vi "Config_LoadCreate.vi"(7 "Config In":path, 8 "error In":errorcluster, 10 "Configuration Cluster":T1={"General"={"Config.ini"=path "", "Default Logging Path"=path ""}, "Hardware"={"Measure Rate (1/s)"=0, "HP DMM VISA"="", "LS 335 VISA"="", "HP DM"={"Range"=enum."Autorange", "Autozero"=FALSE, "Display"=enum."3 1/2 Digit", "Blank LCD"=FALSE}}, "Operation"={"Operation Mode"=enum."Idle-Off", "Status"="", "NewLog?"=FALSE, "OvenWarn"=FALSE}}) -> (0 "error out":errorcluster, 2 "Configuration Cluster Out":T1={"General"={"Config.ini"=path "", "Default Logging Path"=path ""}, "Hardware"={"Measure Rate (1/s)"=0, "HP DMM VISA"="", "LS 335 VISA"="", "HP DM"={"Range"=enum."Autorange", "Autozero"=FALSE, "Display"=enum."3 1/2 Digit", "Blank LCD"=FALSE}}, "Operation"={"Operation Mode"=enum."Idle-Off", "Status"="", "NewLog?"=FALSE, "OvenWarn"=FALSE}})   [LabVIEW 2021]
uses:
  Config_Cluster.ctl
  Mode_Enum.ctl
  <vilib>/Utility/config.llb/Read Key (Path).vi
  <vilib>/Utility/config.llb/NI_LVConfig.lvlib
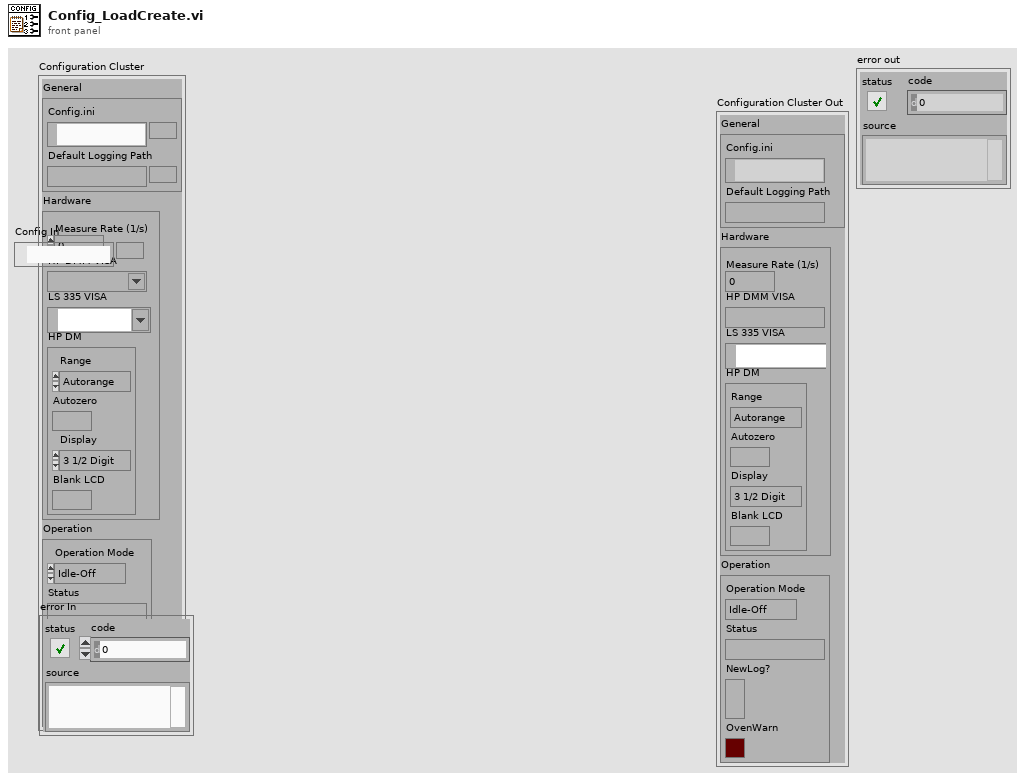
[diagram p1: front panel]
types:
  T1 = typedef "Config_Cluster.ctl" = cluster{"General":cluster{"Config.ini":path, "Default Logging Path":path}, "Hardware":cluster{"Measure Rate (1/s)":i32, "HP DMM VISA":refnum<visa-resource-name>, "LS 335 VISA":refnum<visa-resource-name>, "HP DM":cluster{"Range":enum16{"Autorange", "30mV", "300mV", "3V", "30V"}, "Autozero":bool, "Display":enum16{"3 1/2 Digit", "4 1/2 Digit", "5 1/2 Digit"}, "Blank LCD":bool}}, "Operation":cluster{"Operation Mode":T2, "Status":string, "NewLog?":bool, "OvenWarn":bool}}
  T2 = typedef "Mode_Enum.ctl" = enum16{"OvenNRDY", "Logging", "Idle-Off", "Idle"}
  T3 = typedef "NI_LVConfig.lvlib/Config Data RefNum.ctl" = refnum<k1>
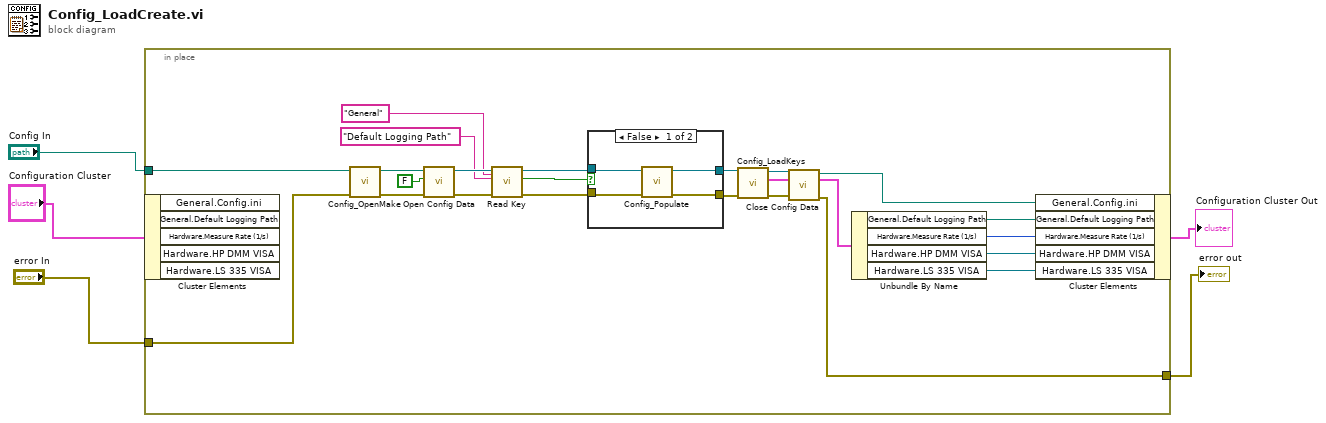
[diagram p0: block diagram]
diagram:
  n1 = in-place {
    in-place-border: "error In" -> [w27]
    in-place-border: "Config In" -> [w28]
    in-place-border: [w8] -> w1
    n2 = in-place-cluster #1("Configuration Cluster") -> ()  [unwired: 5 out]
    n3 = call "Config_OpenMake.vi"("error in (no error)"=w27, "Config Path"=w28) -> ("error out"=w24:errorcluster, "File Path"=w26:path)  [unwired: 8 in]
    n4 = call <vilib>:"Open Config Data.vi"("error in (no error)"=w24, "create file if necessary (T)"=FALSE, "configuration file path"=w26) -> ("error out"=w22:errorcluster, "refnum"=w23:T3)  [unwired: 6 in, 1 out]
    n5 = call-poly <vilib>:"Read Key.vi"("section"="General", "error in (no error)"=w22, "key"="Default Logging Path", "refnum"=w23) -> ("error out"=w18:errorcluster, "found?"=w17:bool, "refnum out"=w19:T3)  [unwired: 4 in, 1 out]
    n6 = case shown="False" w17 {
      tunnel: w18 -> [w31 w33]
      tunnel: w19 -> [w32 w34]
      tunnel: [w30 w33] -> w13
      tunnel: [w29 w34] -> w15
      frame False {
        n7 = call "Config_Populate.vi"("error in (no error)"=w31, "Config Ref In"=w32) -> ("error out"=w30:errorcluster, "refnum out"=w29:T3)  [unwired: 8 in]
      }
      frame True {
      }
    }
    n8 = call "Config_LoadKeys.vi"("error in (no error)"=w13, "Config In"=w15) -> ("error out"=w12:errorcluster, "output cluster"=w11:T1, "refnum out"=w14:T3)  [unwired: 7 in]
    n9 = call <vilib>:"Close Config Data.vi"("error in (no error)"=w12, "refnum"=w14) -> ("error out"=w8:errorcluster, "file path"=w16:path)  [unwired: 8 in]
    n10 = Unbundle By Name(w11) -> ("General.Default Logging Path"=w10:path, "Hardware.Measure Rate (1/s)"=w9:i32, "Hardware.HP DMM VISA"=w7:refnum<visa-resource-name>, "Hardware.LS 335 VISA"=w6:refnum<visa-resource-name>)
    n11 = in-place-cluster #1("General.Config.ini"=w16, "General.Default Logging Path"=w10, "Hardware.Measure Rate (1/s)"=w9, "Hardware.HP DMM VISA"=w7, "Hardware.LS 335 VISA"=w6) -> (→"Configuration Cluster Out":T1)
  }
  "error out" <- w1
